vi "Sysdef.SimpleImport(subSection).vi"(7 "Overwrite Existing?":bool=TRUE, 8 "error in (no error)":errorcluster, 10 "SysDef":T1 {"Tree"."Properties"."Type" items=["K_STRING", "K_BOOL", "K_I32", "K_U32", "K_DOUBLE", "K_U64", "K_VARIANT", "K_DEPENDENTFILE", "K_DEPENDENTNODE", "K_DATASOURCENODE", "K_U16", "K_DBLARR", "K_U32ARR", "K_I32ARR", "K_STRINGARR", "K_DICTIONARY", "K_DICTIONARYARR"]}, 11 "NodeID":u64) -> (0 "error out":errorcluster, 3 "NodeID out":u64)   [LabVIEW 2020, in "ImportExport.lvlib"]
doc: "Uses the NI VeriStand .NET API. to add or edit the Custom Device Hierarchy (Sections, Channels, Waveforms) as well as its Items Properties using the data from the SysDef cluster."
uses:
  ImportExport.lvlib
  <vilib>/NI/NI VeriStand Advanced SysDef API/_Types/SysDef.Export.subSection.ctl
  <vilib>/NI/NI VeriStand Advanced SysDef API/_Types/TreeItem.ctl
  <vilib>/NI/NI VeriStand Advanced SysDef API/_Types/TreeItem.Info.ctl
  <vilib>/NI VeriStand/Custom Device API/Custom Device Channel.ctl
  <vilib>/NI VeriStand/Custom Device API/Custom Device Channel Type.ctl
  <vilib>/NI VeriStand/Custom Device API/Custom Device Waveform.ctl
  <vilib>/NI VeriStand/Custom Device API/Custom Device Waveform DataType.ctl
  <vilib>/NI/NI VeriStand Advanced SysDef API/_Types/TreeItem.Property.ctl
  NationalInstruments.VeriStand.SystemDefinitionAPI
  NationalInstruments.VeriStand.SystemStorage
  <vilib>/NI/NI VeriStand Advanced SysDef API/SysDef API/Advanced System Definition.lvlib
  <vilib>/NI VeriStand/Custom Device API/Custom Device API.lvlib
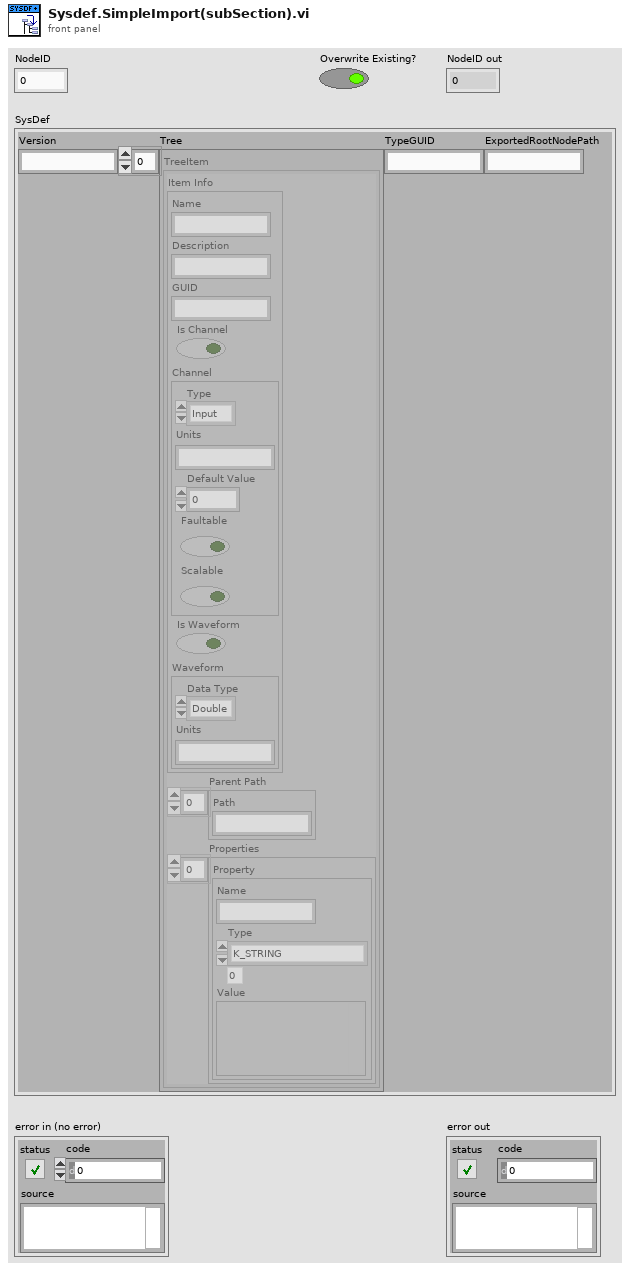
[diagram p1: front panel]
types:
  T1 = typedef "Advanced System Definition.lvlib/SysDef.Export.subSection.ctl" = cluster{"Version":string, "Tree":T2[], "TypeGUID ":string, "ExportedRootNodePath":string}
  T2 = typedef "Advanced System Definition.lvlib/TreeItem.ctl" = cluster{"Item Info":T3, "Parent Path":string[], "Properties":T8[]}
  T3 = typedef "Advanced System Definition.lvlib/TreeItem.Info.ctl" = cluster{"Name":string, "Description":string, "GUID":string, "Is Channel":bool, "Channel":T4, "Is Waveform":bool, "Waveform":T6}
  T4 = typedef "Custom Device API.lvlib/Custom Device Channel.ctl" = cluster{"Type":T5, "Units":string, "Default Value":dbl, "Faultable":bool, "Scalable":bool}
  T5 = typedef "Custom Device API.lvlib/Custom Device Channel Type.ctl" = enum16{"Input", "Output"}
  T6 = typedef "Custom Device API.lvlib/Custom Device Waveform.ctl" = cluster{"Data Type":T7, "Units":string}
  T7 = typedef "Custom Device API.lvlib/Custom Device Waveform DataType.ctl" = enum16{"Double", "Complex Double"}
  T8 = typedef "Advanced System Definition.lvlib/TreeItem.Property.ctl" = cluster{"Name":string, "Type":i32, "Value":variant}
  T9 = typedef "Custom Device API.lvlib/Custom Device Item Ref.ctl" = u64
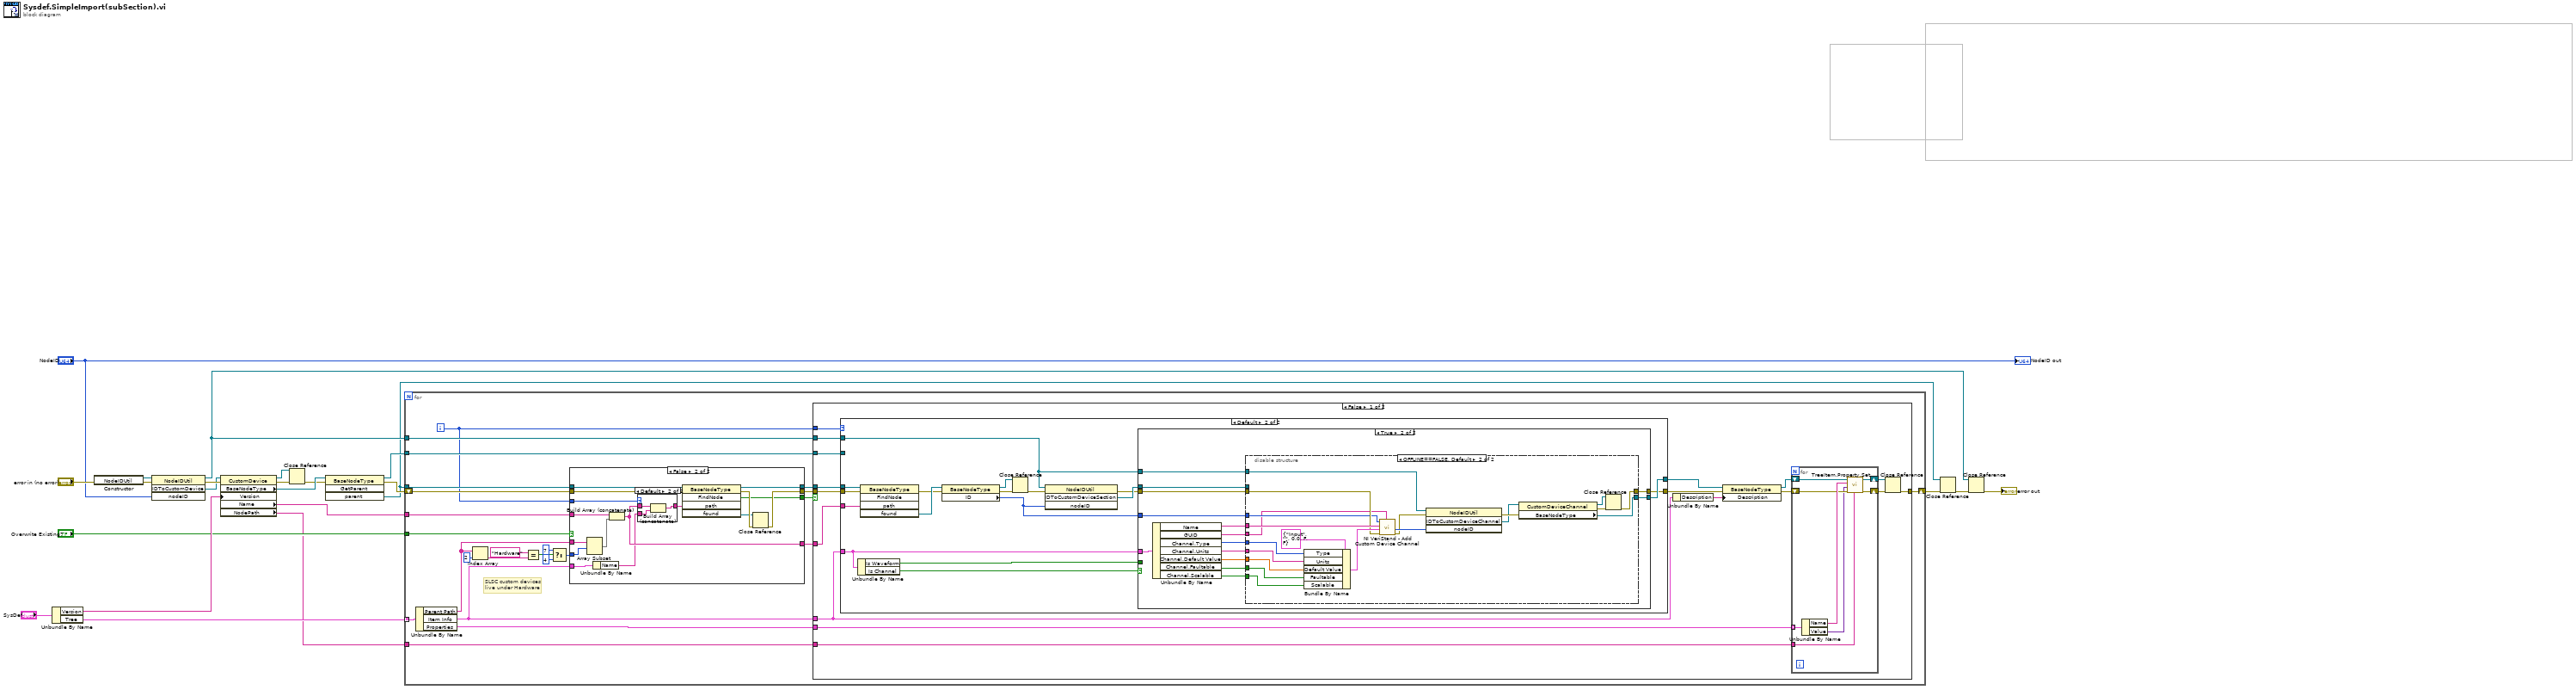
[diagram p0: block diagram]
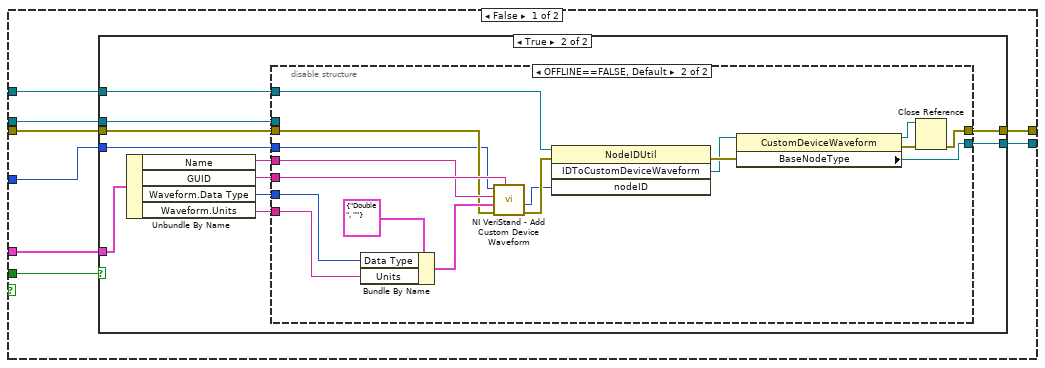
[diagram p3: hidden frame]
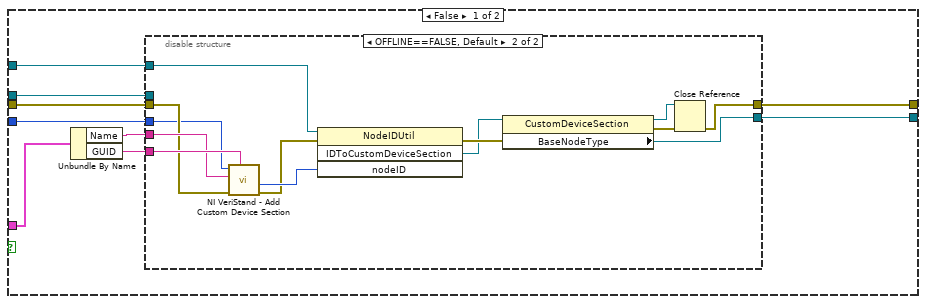
[diagram p4: hidden frame]
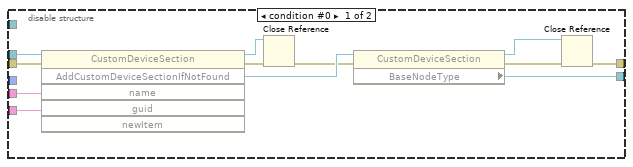
[diagram p5: hidden frame]
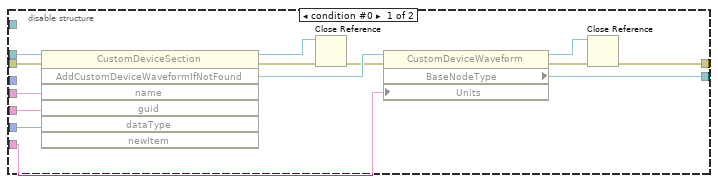
[diagram p6: hidden frame]
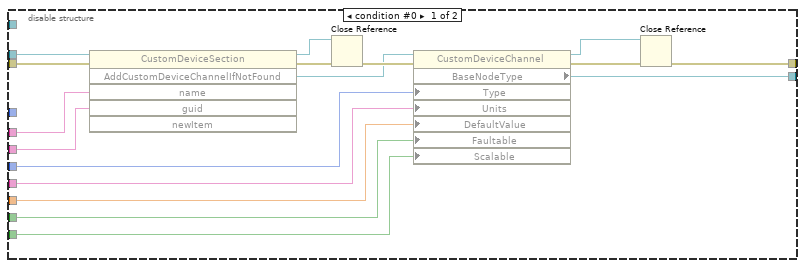
[diagram p7: hidden frame]
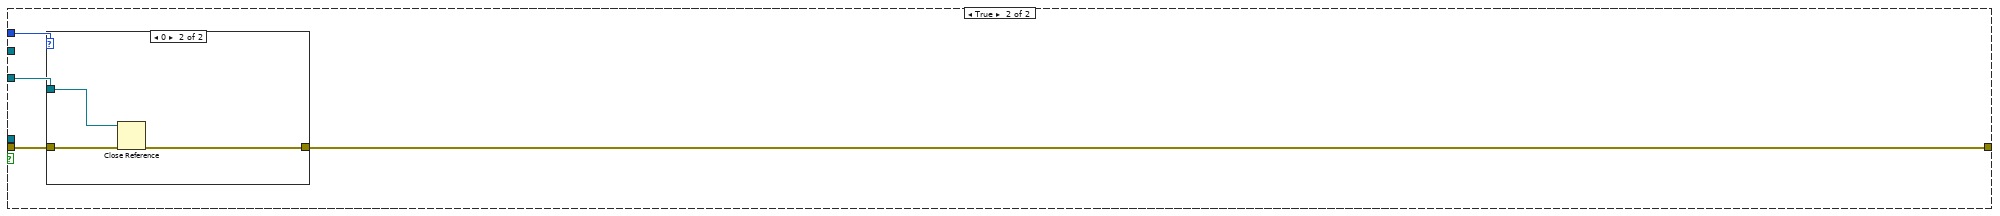
[diagram p8: hidden frame]
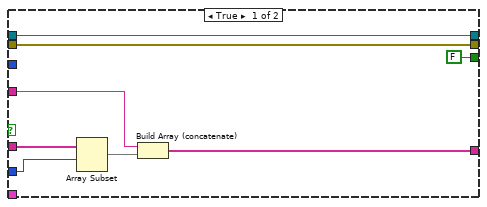
[diagram p10: hidden frame]
diagram:
  n1 = Unbundle By Name("SysDef") -> ("Version"=w21:string, "Tree"=w22:T2[])
  n2 = constructor class="NodeIDUtil"(error in="error in (no error)") -> (reference out=w3:refnum<k24>, error out=w8:errorcluster)  [unwired: 2 in, 1 out]
  n3 = invoke class="NodeIDUtil" method="IDToCustomDevice"(reference=w3, error in=w8, "nodeID"="NodeID") -> (reference out=w14:refnum<k24>, error out=w20:errorcluster, "IDToCustomDevice"=w2:refnum<k24>)  [unwired: 1 in, 1 out]
  n4 = property class="CustomDevice"(reference=w2, error in=w20, "Version"=w21) -> (reference out=w6:refnum<k24>, error out=w5:errorcluster, "BaseNodeType"=w11:refnum<k24>, "Name"=w17:string, "NodePath"=w1:string)
  n5 = Close Reference(reference=w6, error in (no error)=w5) -> (error out=w4:errorcluster)
  n6 = invoke class="BaseNodeType" method="GetParent"(reference=w11, error in=w4) -> (reference out=w18:refnum<k24>, error out=w19:errorcluster, "parent"=w10:refnum<k24>)  [unwired: 2 in, 1 out]
  n7 = for {
    tunnel: w22 -> [w47] mode=indexing
    shift-right: [w45] -> w7
    shift-left: w19 -> [w39]
    tunnel: w18 -> [w44]
    tunnel: w17 -> [w43]
    tunnel: "Overwrite Existing?" -> [w40]
    tunnel: w14 -> [w35]
    tunnel: w10 -> [w34]
    tunnel: w1 -> [w24]
    i -> [w33]
    # "SLSC custom devices\nlive under Hardware"
    n8 = Unbundle By Name(w47) -> ("Parent Path"=w32:string[], "Item Info"=w41:T3, "Properties"=w46:T8[])
    n9 = Index Array(array=w32, index=2) -> (element=w30:string)
    n10 = Equal?(x="Hardware", y=w30) -> (x = y?=w28:bool)
    n11 = Select(t=7 ("index"), s=w28, f=4 ("index")) -> (s? t:f=w25:i32)
    n12 = case shown="False" w40 {
      tunnel: w32 -> [w242 w258]
      tunnel: w43 -> [w240 w256]
      tunnel: [w239 w254] -> w42
      tunnel: w41 -> [_ w255]
      tunnel: w39 -> [w237 w252]
      tunnel: w34 -> [w238 w250]
      tunnel: [w238 w244] -> w38
      tunnel: [w237 w248] -> w37
      tunnel: [FALSE ("FindNode") w247] -> w36
      tunnel: w33 -> [_ w246]
      tunnel: w25 -> [w235 w243]
      frame True {
        n13 = Array Subset(array=w242, index=w235) -> (w241:string[])  [unwired: 1 in]
        n14 = Build Array (concatenate)(w240, w241) -> (w239:string[])
      }
      frame False {
        n15 = Array Subset(array=w258, index=w243) -> (w257:string[])  [unwired: 1 in]
        n16 = Unbundle By Name(w255) -> ("Name"=w253:string)
        n17 = Build Array (concatenate)(w256, w257) -> (w254:string[])
        n18 = case shown="Default" w246 {
          tunnel: w254 -> [w259 w262]
          tunnel: w253 -> [_ w261]
          tunnel: [w259 w260] -> w251
          frame 0 {
          }
          frame Default {
            n19 = Build Array (concatenate)(w262, w261) -> (w260:string[])
          }
        }
        n20 = invoke class="BaseNodeType" method="FindNode"(reference=w250, error in=w252, "path"=w251) -> (reference out=w244:refnum<k24>, error out=w249:errorcluster, "FindNode"=w247:bool, "found"=w245:refnum<k24>)  [unwired: 2 in, 1 out]
        n21 = Close Reference(reference=w245, error in (no error)=w249) -> (error out=w248:errorcluster)
      }
    }
    n22 = case shown="False" w36 {
      tunnel: w46 -> [w64 _]
      tunnel: w35 -> [w63 _]
      tunnel: [w60 w227] -> w45
      tunnel: w33 -> [w59 w230]
      tunnel: w44 -> [w58 w228]
      tunnel: w42 -> [w57 _]
      tunnel: w41 -> [w50 _]
      tunnel: w38 -> [w56 _]
      tunnel: w37 -> [w55 w229]
      tunnel: w24 -> [w48 _]
      frame False {
        n23 = case shown="Default" w59 {
          tunnel: w55 -> [w65 w81]
          tunnel: [w65 w73] -> w54
          tunnel: [w66 w74] -> w53
          tunnel: w56 -> [_ w69]
          tunnel: w57 -> [_ w83]
          tunnel: w50 -> [_ w75]
          tunnel: w63 -> [_ w67]
          tunnel: w58 -> [w66 _]
          frame 0 {
          }
          frame Default {
            n24 = Unbundle By Name(w75) -> ("Is Waveform"=w72:bool, "Is Channel"=w76:bool)
            n25 = invoke class="BaseNodeType" method="FindNode"(reference=w69, error in=w81, "path"=w83) -> (error out=w80:errorcluster, "found"=w82:refnum<k24>)  [unwired: 2 in, 3 out]
            n26 = property class="BaseNodeType"(reference=w82, error in=w80) -> (reference out=w70:refnum<k24>, error out=w79:errorcluster, "ID"=w68:u64)
            n27 = Close Reference(reference=w70, error in (no error)=w79) -> (error out=w71:errorcluster)
            n28 = invoke class="NodeIDUtil" method="IDToCustomDeviceSection"(reference=w67, error in=w71, "nodeID"=w68) -> (error out=w77:errorcluster, "IDToCustomDeviceSection"=w78:refnum<k24>)  [unwired: 1 in, 2 out]
            n29 = case shown="True" w76 {
              tunnel: w78 -> [w90 w177]
              tunnel: w77 -> [w89 w174]
              tunnel: w75 -> [w87 w170]
              tunnel: [w88 w173] -> w74
              tunnel: [w86 w171] -> w73
              tunnel: w72 -> [w91 _]
              tunnel: w68 -> [w85 w169]
              tunnel: w67 -> [w84 w168]
              frame False {
                n30 = case shown="True" w91 {
                  tunnel: w90 -> [w99 w136]
                  tunnel: w89 -> [w100 w135]
                  tunnel: [w96 w129] -> w88
                  tunnel: [w95 w131] -> w86
                  tunnel: w87 -> [w98 w134]
                  tunnel: w85 -> [w93 w127]
                  tunnel: w84 -> [w92 w126]
                  frame False {
                    n31 = Unbundle By Name(w98) -> ("Name"=w94:string, "GUID"=w97:string)
                    n32 = disable-structure shown="OFFLINE==FALSE, Default" {
                      disable-tunnel: w100 -> [w110 w123]
                      disable-tunnel: w99 -> [w109 _]
                      disable-tunnel: w97 -> [w108 w125]
                      disable-tunnel: [w106 w114] -> w96
                      disable-tunnel: [w102 w113] -> w95
                      disable-tunnel: w94 -> [w101 w124]
                      disable-tunnel: w93 -> [_ w122]
                      disable-tunnel: w92 -> [_ w115]
                      frame condition #0 {
                        n33 = invoke class="CustomDeviceSection" method="AddCustomDeviceSectionIfNotFound"(reference=w109, error in=w110, "name"=w101, "guid"=w108) -> (reference out=w111:refnum<k24>, error out=w112:errorcluster, "AddCustomDeviceSectionIfNotFound"=w107:refnum<k24>)  [unwired: 2 in, 3 out]
                        n34 = Close Reference(reference=w111, error in (no error)=w112) -> (error out=w105:errorcluster)
                        n35 = property class="CustomDeviceSection"(reference=w107, error in=w105) -> (reference out=w104:refnum<k24>, error out=w103:errorcluster, "BaseNodeType"=w106:refnum<k24>)
                        n36 = Close Reference(reference=w104, error in (no error)=w103) -> (error out=w102:errorcluster)
                      }
                      frame condition #1 (active) {
                        n37 = call <vilib>:"NI VeriStand - Add Custom Device Section.vi"("GUID (Default Section)"=w125, "error in (no error)"=w123, "Section Name"=w124, "Parent Ref in"=w122) -> ("error out"=w116:errorcluster, "Section Ptr"=w117:T9)  [unwired: 4 in, 2 out]
                        n38 = invoke class="NodeIDUtil" method="IDToCustomDeviceSection"(reference=w115, error in=w116, "nodeID"=w117) -> (error out=w121:errorcluster, "IDToCustomDeviceSection"=w120:refnum<k24>)  [unwired: 1 in, 2 out]
                        n39 = property class="CustomDeviceSection"(reference=w120, error in=w121) -> (reference out=w119:refnum<k24>, error out=w118:errorcluster, "BaseNodeType"=w114:refnum<k24>)
                        n40 = Close Reference(reference=w119, error in (no error)=w118) -> (error out=w113:errorcluster)
                      }
                    }
                  }
                  frame True {
                    n41 = Unbundle By Name(w134) -> ("Name"=w128:string, "GUID"=w133:string, "Waveform.Data Type"=w132:T7, "Waveform.Units"=w130:string)
                    n42 = disable-structure shown="OFFLINE==FALSE, Default" {
                      disable-tunnel: w136 -> [w146 _]
                      disable-tunnel: w135 -> [w145 w161]
                      disable-tunnel: w133 -> [w144 w167]
                      disable-tunnel: w132 -> [w143 w165]
                      disable-tunnel: [w140 w155] -> w131
                      disable-tunnel: w130 -> [w139 w164]
                      disable-tunnel: [w138 w154] -> w129
                      disable-tunnel: w128 -> [w137 w162]
                      disable-tunnel: w127 -> [_ w152]
                      disable-tunnel: w126 -> [_ w151]
                      frame condition #0 {
                        n43 = invoke class="CustomDeviceSection" method="AddCustomDeviceWaveformIfNotFound"(reference=w146, error in=w145, "name"=w137, "guid"=w144, "dataType"=w143) -> (reference out=w149:refnum<k24>, error out=w150:errorcluster, "AddCustomDeviceWaveformIfNotFound"=w148:refnum<k24>)  [unwired: 2 in, 4 out]
                        n44 = Close Reference(reference=w149, error in (no error)=w150) -> (error out=w147:errorcluster)
                        n45 = property class="CustomDeviceWaveform"(reference=w148, error in=w147, "Units"=w139) -> (reference out=w142:refnum<k24>, error out=w141:errorcluster, "BaseNodeType"=w138:refnum<k24>)
                        n46 = Close Reference(reference=w142, error in (no error)=w141) -> (error out=w140:errorcluster)
                      }
                      frame condition #1 (active) {
                        n47 = Bundle By Name(cluster=T6 {"Data Type"=enum."Double", "Units"=""} ("Waveform"), "Data Type"=w165, "Units"=w164) -> (w163:T6)
                        n48 = call <vilib>:"NI VeriStand - Add Custom Device Waveform.vi"("GUID (Default Waveform)"=w167, "error in (no error)"=w161, "Waveform"=w163, "Waveform Name"=w162, "Parent Ref in"=w152) -> ("error out"=w156:errorcluster, "Waveform Ref"=w153:T9)  [unwired: 3 in, 2 out]
                        n49 = invoke class="NodeIDUtil" method="IDToCustomDeviceWaveform"(reference=w151, error in=w156, "nodeID"=w153) -> (error out=w160:errorcluster, "IDToCustomDeviceWaveform"=w159:refnum<k24>)  [unwired: 1 in, 2 out]
                        n50 = property class="CustomDeviceWaveform"(reference=w159, error in=w160) -> (reference out=w158:refnum<k24>, error out=w157:errorcluster, "BaseNodeType"=w154:refnum<k24>)
                        n51 = Close Reference(reference=w158, error in (no error)=w157) -> (error out=w155:errorcluster)
                      }
                    }
                  }
                }
              }
              frame True {
                n52 = Unbundle By Name(w170) -> ("Name"=w172:string, "GUID"=w176:string, "Channel.Type"=w175:T5, "Channel.Units"=w181:string, "Channel.Default Value"=w180:dbl, "Channel.Faultable"=w179:bool, "Channel.Scalable"=w178:bool)
                n53 = disable-structure shown="OFFLINE==FALSE, Default" {
                  disable-tunnel: w181 -> [w197 w215]
                  disable-tunnel: w180 -> [w196 w214]
                  disable-tunnel: w179 -> [w195 w213]
                  disable-tunnel: w178 -> [w194 w212]
                  disable-tunnel: w177 -> [w193 _]
                  disable-tunnel: w176 -> [w192 w199]
                  disable-tunnel: w175 -> [w191 w216]
                  disable-tunnel: w174 -> [w189 w210]
                  disable-tunnel: [w188 w206] -> w173
                  disable-tunnel: w172 -> [w187 w218]
                  disable-tunnel: [w186 w200] -> w171
                  disable-tunnel: w169 -> [_ w209]
                  disable-tunnel: w168 -> [_ w207]
                  frame condition #0 {
                    n54 = invoke class="CustomDeviceSection" method="AddCustomDeviceChannelIfNotFound"(reference=w193, error in=w189, "name"=w187, "guid"=w192) -> (reference out=w182:refnum<k24>, error out=w185:errorcluster, "AddCustomDeviceChannelIfNotFound"=w183:refnum<k24>)  [unwired: 2 in, 3 out]
                    n55 = Close Reference(reference=w182, error in (no error)=w185) -> (error out=w198:errorcluster)
                    n56 = property class="CustomDeviceChannel"(reference=w183, error in=w198, "Type"=w191, "Units"=w197, "DefaultValue"=w196, "Faultable"=w195, "Scalable"=w194) -> (reference out=w190:refnum<k24>, error out=w184:errorcluster, "BaseNodeType"=w188:refnum<k24>)
                    n57 = Close Reference(reference=w190, error in (no error)=w184) -> (error out=w186:errorcluster)
                  }
                  frame condition #1 (active) {
                    n58 = Bundle By Name(cluster=T4 {"Type"=enum."Input", "Units"="", "Default Value"=0.0, "Faultable"=FALSE, "Scalable"=FALSE} ("Channel"), "Type"=w216, "Units"=w215, "Default Value"=w214, "Faultable"=w213, "Scalable"=w212) -> (w211:T4)
                    n59 = call <vilib>:"NI VeriStand - Add Custom Device Channel.vi"("GUID (Default Channel)"=w199, "error in (no error)"=w210, "Channel"=w211, "Channel Name"=w218, "Parent Ref in"=w209) -> ("error out"=w205:errorcluster, "Channel Ref"=w208:T9)  [unwired: 3 in, 2 out]
                    n60 = invoke class="NodeIDUtil" method="IDToCustomDeviceChannel"(reference=w207, error in=w205, "nodeID"=w208) -> (error out=w204:errorcluster, "IDToCustomDeviceChannel"=w203:refnum<k24>)  [unwired: 1 in, 2 out]
                    n61 = property class="CustomDeviceChannel"(reference=w203, error in=w204) -> (reference out=w202:refnum<k24>, error out=w201:errorcluster, "BaseNodeType"=w206:refnum<k24>)
                    n62 = Close Reference(reference=w202, error in (no error)=w201) -> (error out=w200:errorcluster)
                  }
                }
              }
            }
          }
        }
        n63 = Unbundle By Name(w50) -> ("Description"=w49:string)
        n64 = property class="BaseNodeType"(reference=w53, error in=w54, "Description"=w49) -> (reference out=w51:refnum<k24>, error out=w52:errorcluster)
        n65 = for {
          shift-right: [w226] -> w61
          shift-left: w52 -> [w221]
          tunnel: w64 -> [w224] mode=indexing
          shift-right: [w223] -> w62
          shift-left: w51 -> [w225]
          tunnel: w48 -> [w219]
          n66 = Unbundle By Name(w224) -> ("Name"=w222:string, "Value"=w220:variant)
          n67 = call <vilib>:"TreeItem.Property.Set.vi"("Custom Device Path"=w219, "error in (no error)"=w221, "Value"=w220, "Property Name"=w222, "BaseNodeType"=w225) -> ("error out"=w226:errorcluster, "BaseNodeType"=w223:refnum<k24>)  [unwired: 4 in, 1 out]
        }
        n68 = Close Reference(reference=w62, error in (no error)=w61) -> (error out=w60:errorcluster)
      }
      frame True {
        n69 = case shown="0" w230 {
          tunnel: w229 -> [w231 w234]
          tunnel: [w231 w233] -> w227
          tunnel: w228 -> [_ w232]
          frame Default {
          }
          frame 0 {
            n70 = Close Reference(reference=w232, error in (no error)=w234) -> (error out=w233:errorcluster)
          }
        }
      }
    }
  }
  n71 = Close Reference(reference=w10, error in (no error)=w7) -> (error out=w15:errorcluster)
  n72 = Close Reference(reference=w14, error in (no error)=w15) -> (error out=→"error out":errorcluster)
  "NodeID out" <- "NodeID"
